vi "AbortHardware.vi"(8 "error in (no error)":errorcluster, 11 "NewportXPS in":refnum<class "NewportXPS.lvclass">) -> (0 "error out":errorcluster)   [LabVIEW 2020]
uses:
  NewportXPS.lvclass
  C:/GEECS/Developers Version/source/Device Drivers/BaseDriver/BaseDriver.lvclass
  C:/GEECS/Developers Version/source/Device Drivers/NewportXPS/NewportXPS.lvclass
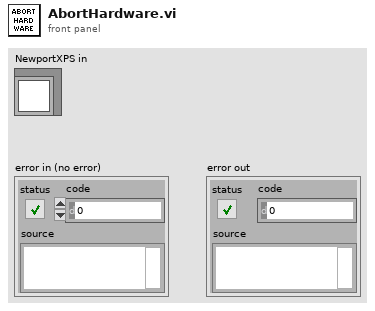
[diagram p1: front panel]
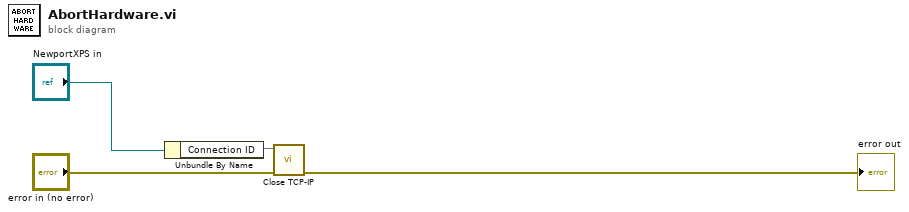
[diagram p0: block diagram]
diagram:
  n1 = Unbundle By Name("NewportXPS in") -> ("Connection ID"=w4)
  n2 = call "Close TCP-IP.vi"("error in (no error)"="error in (no error)", "connection ID in"=w4) -> ("Error out"=→"error out":errorcluster)  [unwired: 9 in]
